vi "PH_SHS_Analysis_Calibrator.save calibration data.vi"(0 "i ref in":refnum<vi>, 5 "error in (no error)":errorcluster) -> (14 "i ref out":refnum<vi>, 19 "error out":errorcluster)   [LabVIEW 2014, in "PH_SHS_Analysis_Calibrator.lvlib"]
doc: "This VI saves the calibration data."
uses:
  PH_SHS_Analysis_Calibrator.lvlib
  PH_SHS_Analysis_Calibrator.Analysis Calibration Data.ctl
  CSlibraries-extern/shs/SHS_Common/SHSReference.ctl
  CSlibraries-extern/shs/SHS_Common/ReferencePoint.ctl
  CSlibraries-extern/shs/SHS_Common/Rectangle.ctl
  CSlibraries-extern/shs/SHS_Common/Point.ctl
  PH_Basics/PH_Img_BaseClass/PH_Img_BaseClass.lvlib
  CSlibraries-extern/shs/SHS_Common/SHS_Common.lvlib
panel:
  in  "SHS Analysis Calibration data":T1
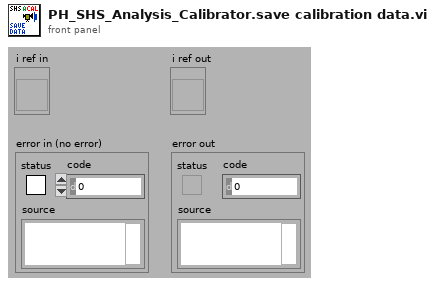
[diagram p1: front panel]
types:
  T1 = typedef "PH_SHS_Analysis_Calibrator.lvlib/PH_SHS_Analysis_Calibrator.Analysis Calibration Data.ctl" = cluster{"Date":string, "Time":string, "Cam Settings":cluster{"Cam ID":string, "Gain":dbl, "Brightness":dbl, "Shutter":dbl, "Cam Error":bool, "Mode":i32}, "SHS Reference Result":T2, "Pixel Size":dbl, "MLA Pitch":dbl, "Method":enum16{"automatic", "manual"}, "Calibration Data calculated":bool, "No Problems at calculation?":bool, "error out":errorcluster}
  T2 = typedef "SHS_Common.lvlib/SHSReference.ctl" = cluster{"Reference":T3[][], "Lens Array Pitch [px]":dbl}
  T3 = typedef "SHS_Common.lvlib/ReferencePoint.ctl" = cluster{"Rect":T4, "Point":T5}
  T4 = typedef "SHS_Common.lvlib/Rectangle.ctl" = cluster{"Left":i32, "Top":i32, "Right":i32, "Bottom":i32}
  T5 = typedef "SHS_Common.lvlib/Point.ctl" = cluster{"x":dbl, "y":dbl, "valid?":bool, "weight":dbl}
  T6 = typedef "PH_SHS_Analysis_Calibrator.lvlib/PH_SHS_Analysis_Calibrator.i attribute.ctl" = cluster{"GUI Refs":cluster{"Available Cams":refnum<vi>, "OK":refnum<vi>, "Skip":refnum<vi>, "Repeat":refnum<vi>, "Cancel":refnum<vi>, "Dialog":refnum<vi>, "Enough Images?":refnum<vi>}, "Cam instances":string[], "Status":cluster{"#":i32, "Data calculated":bool, "Wanted #":i32}, "IMAQ Image Array":T7[], "Pixel Size [µm]":dbl, "MLA Pitch [µm]":dbl, "Method":enum16{"automatic", "manual"}, "Enough Images?":bool, "SHS Reference Result":T2, "Calculation Error":errorcluster}
  T7 = typedef "IMAQ Image.ctl" = refnum<image>
  T8 = typedef "PH_Img_BaseClass.lvlib/PH_Img_BaseClass.i attribute.ctl" = cluster{"GUI Refs":T9, "Timeout Image [ms]":i32, "Default Periodic Period [ms]":i32, "Camera":cluster{"Instancename":string, "Notifier":refnum<notifier>}, "Palette":T10, "Cam Settings":cluster{"Cam ID":string, "Gain":dbl, "Brightness":dbl, "Shutter":dbl, "Cam Info Failure":bool, "Mode":i32}}
  T9 = typedef "PH_Img_BaseClass.lvlib/PH_Img_BaseClass.GUI Refs.ctl" = cluster{"Timeout":refnum<vi>, "Image":refnum<vi>, "Palette":refnum<vi>, "Timeout Set":refnum<vi>}
  T10 = typedef "PH_Img_BaseClass.lvlib/PH_Img_BaseClass.Palette.ctl" = i32
  T11 = cluster{"Cam ID":string, "Gain":dbl, "Brightness":dbl, "Shutter":dbl, "Cam Info Failure":bool, "Mode":i32}
  T12 = enum16{"open", "replace", "create", "open or create", "replace or create", "replace or create with confirmation"}
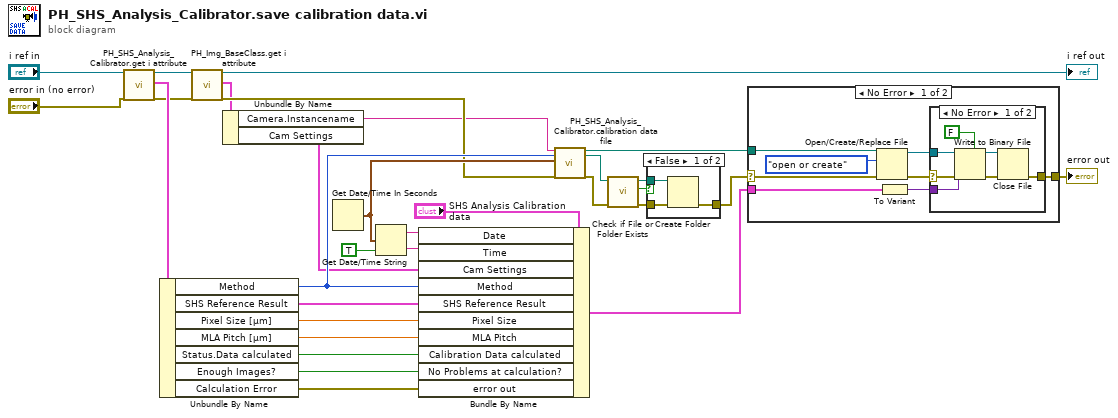
[diagram p0: block diagram]
diagram:
  n1 = call "PH_SHS_Analysis_Calibrator.get i attribute.vi"("i ref in"="i ref in", "error in (no error)"="error in (no error)") -> ("i ref out"=w5:refnum<vi>, "i attribute"=w29:T6, "error out"=w14:errorcluster)  [unwired: 15 in]
  n2 = Unbundle By Name(w29) -> ("Method"=w15:enum16{"automatic", "manual"}, "SHS Reference Result"=w25:T2, "Pixel Size [µm]"=w24:dbl, "MLA Pitch [µm]"=w23:dbl, "Status.Data calculated"=w22:bool, "Enough Images?"=w21:bool, "Calculation Error"=w20:errorcluster)
  n3 = call "PH_Img_BaseClass.get i attribute.vi"("i ref in"=w5, "error in (no error)"=w14) -> ("i ref out"=→"i ref out":refnum<vi>, "i attribute"=w3:T8, "error out"=w6:errorcluster)  [unwired: 15 in]
  n4 = Unbundle By Name(w3) -> ("Camera.Instancename"=w2:string, "Cam Settings"=w1:T11)
  n5 = Get Date/Time In Seconds() -> (seconds since 1Jan1904=w16:timestamp)
  n6 = Get Date/Time String(seconds (now)=w16, want seconds? (F)=TRUE) -> (date string=w18:string, time string=w17:string)  [unwired: 1 in]
  n7 = Bundle By Name(cluster="SHS Analysis Calibration data", "Date"=w18, "Time"=w17, "Cam Settings"=w1, "Method"=w15, "SHS Reference Result"=w25, "Pixel Size"=w24, "MLA Pitch"=w23, "Calibration Data calculated"=w22, "No Problems at calculation?"=w21, "error out"=w20) -> (w19:T1)
  n8 = call "PH_SHS_Analysis_Calibrator.calibration data file.vi"("Camera Instance"=w2, "Method"=w15, "Time of Calibration Data saving"=w16, "error in"=w6) -> ("File to save SHS Analysis Calibration Data in"=w7:path, "Directory path to save  SHS Analysis Calibration Data in"=w8:path, "error out"=w11:errorcluster)  [unwired: 8 in, 5 out]
  n9 = call <vilib>:"Check if File or Folder Exists.vi"("error in (no error)"=w11, "path"=w8) -> ("error out"=w12:errorcluster, "file or folder exists?"=w9:bool, "dup path"=w13:path)  [unwired: 7 in]
  n10 = case shown="False" w9 {
    tunnel: w12 -> [w33 w35]
    tunnel: w13 -> [w34 _]
    tunnel: [w32 w35] -> w10
    frame False {
      n11 = Create Folder(path (use dialog)=w34, error in=w33) -> (error out=w32:errorcluster)  [unwired: 1 in, 2 out]
    }
    frame True {
    }
  }
  n12 = case shown="No Error" w10 {
    selector: w10 -> [w39 w52]
    tunnel: [w43 w52] -> w26
    tunnel: w7 -> [w40 _]
    tunnel: w19 -> [w41 _]
    frame No Error {
      n13 = Open/Create/Replace File(file path (use dialog)=w40, error in=w39, operation (0:open)=T12."open or create") -> (refnum out=w38:refnum<file>, error out=w36:errorcluster)  [unwired: 3 in, 1 out]
      n14 = To Variant(anything=w41) -> (Variant=w42:variant)
      n15 = case shown="No Error" w36 {
        selector: w36 -> [w44 w51]
        tunnel: [w48 w51] -> w43
        tunnel: w42 -> [w47 _]
        tunnel: w38 -> [w45 _]
        frame No Error {
          n16 = Write to Binary File(file (use dialog)=w45, data=w47, error in=w44, 5:FALSE ("prepend array or string size? (T)")) -> (refnum out=w49:refnum<file>, error out=w50:errorcluster)  [unwired: 2 in, 1 out]
          n17 = Close File(refnum=w49, error in=w50) -> (error out=w48:errorcluster)  [unwired: 1 out]
        }
        frame Error {
        }
      }
    }
    frame Error {
    }
  }
  "error out" <- w26
